vi "SetAOs.vi"(0 "FPGA API in":refnum<class "FPGA API Concrete.lvclass">, 5 "ao":dbl[](array[numeric]), 11 "error in (no error)":errorcluster) -> (4 "FPGA API out":refnum<class "FPGA API Concrete.lvclass">, 15 "error out":errorcluster)   [LabVIEW 2019, in "FPGA API Concrete.lvclass"]
uses:
  FPGA API Concrete.lvclass
  FPGA API Concrete.lvclass/FPGA API Concrete.ctl
  <vilib>/Utility/error.llb/Error Cluster From Error Code.vi
  <vilib>/rvi/errors/niLvFpgaAdjustHostInterfaceError.vi
  <vilib>/rvi/interface/nirviReadWriteControl/nirviReadWriteControl.xnode
  FPGA Ref.ctl
  NiFpgaLv.dll
  <vilib>/rvi/interface/Simulation/niFpgaSimulationCallBeginRW.vi
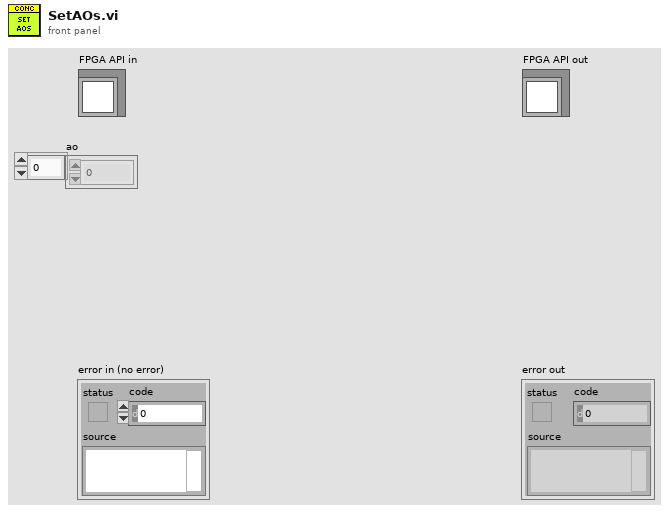
[diagram p1: front panel]
types:
  T1 = typedef "FPGA API Concrete.lvclass/FPGA Ref.ctl" = refnum<k20>
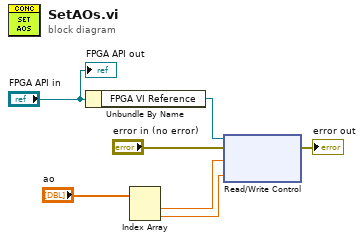
[diagram p0: block diagram]
diagram:
  n1 = Unbundle By Name("FPGA API in") -> ("FPGA VI Reference"=w6:T1)
  n2 = Index Array(array="ao") -> (element #1=w2:dbl, element #2=w1:dbl)  [unwired: 2 in]
  n3 = xnode "Read/Write Control"("FPGA VI Reference In"=w6, "error in"="error in (no error)", "Mod5/AO0"=w2, "Mod5/AO1"=w1) -> ("error out"=→"error out":errorcluster)  [unwired: 1 out]
  "FPGA API out" <- "FPGA API in"
